vi "crit4.vi"(0 "Array":dbl[](array[numeric])) -> (1 "Valid":bool, 2 "trend":dbl[](array[numeric]))   [LabVIEW 2010]
uses:
  <vilib>/addons/Time Series Analysis/Series Preprocess.llb/TSA Detrend (Array).vi
  <vilib>/addons/_Advanced Signal Processing/NI_AdvSigProcTSA.lvlib
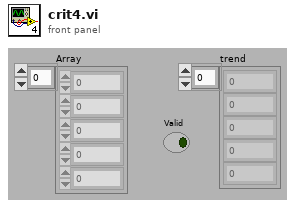
[diagram p1: front panel]
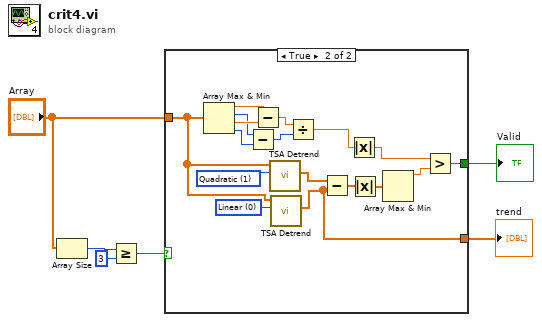
[diagram p0: block diagram]
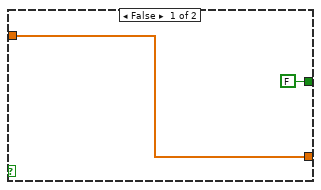
[diagram p2: hidden frame]
diagram:
  n1 = Array Size(array="Array") -> (size(s)=w3:i32)
  n2 = Greater Or Equal?(x=w3, y=3) -> (x >= y?=w1:bool)
  n3 = case shown="True" w1 {
    tunnel: [w8 w25] -> w6
    tunnel: [FALSE w21] -> w5
    tunnel: "Array" -> [w8 w9]
    frame False {
    }
    frame True {
      w12 = u16 1 items=["Linear", "Quadratic", "Cubic", "N-polynomial", "Exponential"] ("method")
      w15 = u16 0 items=["Linear", "Quadratic", "Cubic", "N-polynomial", "Exponential"] ("method")
      n4 = Array Max & Min(array=w9) -> (max value=w14:dbl, max index (indices)=w11:i32, min value=w13:dbl, min index (indices)=w10:i32)
      n5 = Subtract(x=w11, y=w10) -> (x-y=w17:i32)
      n6 = Subtract(x=w14, y=w13) -> (x-y=w16:dbl)
      n7 = call-poly <vilib>:"TSA Detrend.vi"("method"=w12, "Xt"=w9) -> ("trend"=w18:dbl[])  [unwired: 7 in, 2 out]
      n8 = call-poly <vilib>:"TSA Detrend.vi"("method"=w15, "Xt"=w9) -> ("trend"=w25:dbl[])  [unwired: 7 in, 2 out]
      n9 = Divide(x=w16, y=w17) -> (x/y=w23:dbl)
      n10 = Subtract(x=w18, y=w25) -> (x-y=w22:dbl[])
      n11 = Absolute Value(x=w23) -> (abs(x)=w24:dbl)
      n12 = Absolute Value(x=w22) -> (abs(x)=w19:dbl[])
      n13 = Array Max & Min(array=w19) -> (max value=w20:dbl)  [unwired: 3 out]
      n14 = Greater?(x=w24, y=w20) -> (0:w21:bool)
    }
  }
  "trend" <- w6
  "Valid" <- w5
